vi "lidarAngle.vi"(11 "points":cluster{dbl, dbl}[](array[cluster])) -> (0 "detectedAngle (deg)":dbl, 1 "plot":cluster{dbl[], dbl[]}, 3 "correctedPoints":cluster{dbl, dbl}[](array[cluster]))   [LabVIEW 2015]
panel:
  out "Waveform Graph":dbl[](graph)
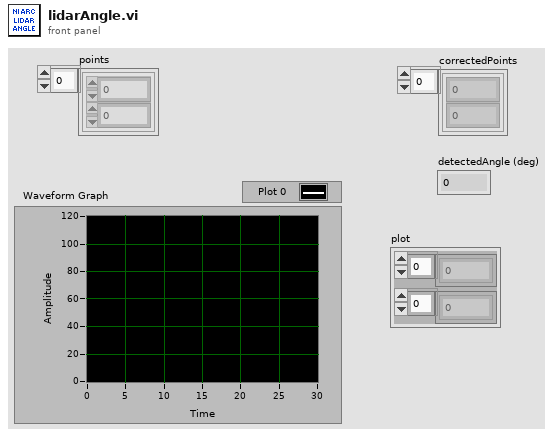
[diagram p1: front panel]
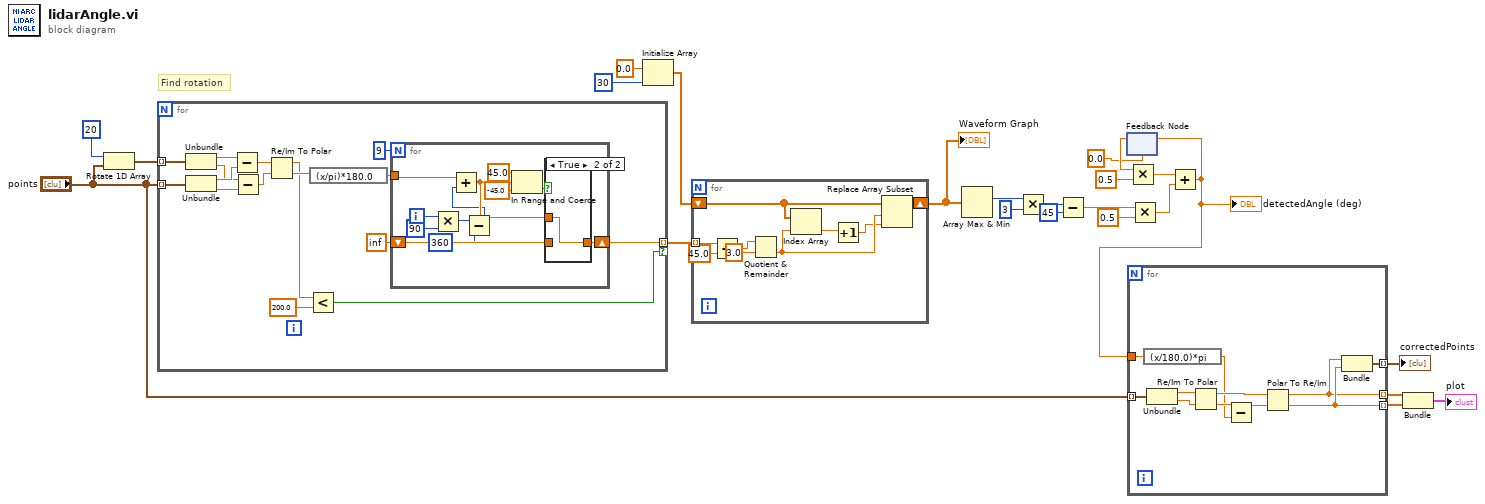
[diagram p0: block diagram]
diagram:
  # "Find rotation"
  n1 = Rotate 1D Array(1:"points", 2:20 ("n")) -> (0:w23:cluster{dbl, dbl}[])
  n2 = for {
    tunnel: w23 -> [w40] mode=indexing
    tunnel: "points" -> [w39] mode=indexing
    tunnel: [w28] -> w22 mode=indexing if=w25
    n3 = Unbundle(w40) -> (w38:dbl, w36:dbl)
    n4 = Unbundle(w39) -> (w37:dbl, w35:dbl)
    n5 = Subtract(x=w38, y=w37) -> (x-y=w34:dbl)
    n6 = Subtract(x=w36, y=w35) -> (x-y=w33:dbl)
    n7 = Re/Im To Polar(2:w33, 3:w34) -> (0:w31:dbl, 1:w27:dbl)
    n8 = Less?(x=w27, y=200.0) -> (x < y?=w25:bool)
    n9 = expression code="(x/pi)*180.0" ("radians to degrees")(w31) -> (w30:dbl)
    n10 = for {
      N: 9 -> [_]
      tunnel: w30 -> [w50]
      shift-right: [w45] -> w28
      shift-left: inf -> [w44]
      i -> [w52]
      n11 = Multiply(x=w52, y=90) -> (x*y=w43:i32)
      n12 = Subtract(x=w43, y=360) -> (x-y=w41:i32)
      n13 = Add(x=w50, y=w41) -> (x+y=w46:dbl)
      n14 = In Range and Coerce(upper limit=45.0, x=w46, lower limit=-45.0) -> (In Range?=w47:bool)  [unwired: 1 out]
      n15 = case shown="True" w47 {
        tunnel: w46 -> [_ w54]
        tunnel: [w53 w54] -> w45
        tunnel: w44 -> [w53 _]
        frame False {
        }
        frame True {
        }
      }
    }
  }
  n16 = Initialize Array(0.0 ("element"), 30 ("dimension size")) -> (w19:dbl[])
  n17 = for {
    tunnel: w22 -> [w57] mode=indexing
    shift-right: [w58] -> w1
    shift-left: w19 -> [w60]
    n18 = Add(x=w57, y=45.0) -> (x+y=w55:dbl)
    n19 = Quotient & Remainder(x=w55, y=3.0) -> (floor(x/y)=w61:dbl)  [unwired: 1 out]
    n20 = Index Array(array=w60, index=w61) -> (element=w62:dbl)
    n21 = Increment(x=w62) -> (x+1=w59:dbl)
    n22 = Replace Array Subset(array=w60, new element=w59, index=w61) -> (w58:dbl[])
  }
  "Waveform Graph" <- w1
  n23 = Array Max & Min(array=w1) -> (max index (indices)=w18:i32)  [unwired: 3 out]
  n24 = Multiply(x=w18, y=3) -> (x*y=w16:i32)
  n25 = Subtract(x=w16, y=45) -> (x-y=w14:dbl)
  n26 = feedback #1(0.0 ("y")) -> (w12:dbl)
  n27 = Multiply(x=w12, y=0.5) -> (x*y=w9:dbl)
  n28 = Multiply(x=w14, y=0.5) -> (x*y=w8:dbl)
  n29 = Add(x=w9, y=w8) -> (x+y=w7:dbl)
  "detectedAngle (deg)" <- w7
  n30 = feedback-in #1(w7) -> ()
  n31 = for {
    tunnel: "points" -> [w74] mode=indexing
    tunnel: w7 -> [w68]
    tunnel: [w65] -> w4 mode=indexing
    tunnel: [w66] -> w3 mode=indexing
    tunnel: [w64] -> w5 mode=indexing
    n32 = expression code="(x/180.0)*pi" ("degrees to radians")(w68) -> (w67:dbl)
    n33 = Unbundle(w74) -> (w73:dbl, w72:dbl)
    n34 = Re/Im To Polar(2:w72, 3:w73) -> (0:w71:dbl, 1:w69:dbl)
    n35 = Subtract(x=w71, y=w67) -> (x-y=w70:dbl)
    n36 = Polar To Re/Im(2:w70, 3:w69) -> (0:w66:dbl, 1:w65:dbl)
    n37 = Bundle(w65, w66) -> (w64:cluster{dbl, dbl})  [unwired: 1 in]
  }
  "correctedPoints" <- w5
  n38 = Bundle(w4, w3) -> (→"plot":cluster{dbl[], dbl[]})  [unwired: 1 in]
